vi "Color Sensor V3 Get CIE Yxy.vi"(8 "error in (no error)":errorcluster, 11 "ColorSensorDevRef":T1={"I2CDevRef"={"DevStatus"={"status"=FALSE, "code"=0, "source"=""}, "Device Address"=0, "Handle"=0, "I2C Bus"=enum."Invalid"}} {"I2CDevRef"."Device Address" format="%.0x"}) -> (0 "error out":errorcluster, 2 "CIE Yxy":cluster{"Yx":dbl, "Yy":dbl}, 3 "ColorSensorDevRef out":T1={"I2CDevRef"={"DevStatus"={"status"=FALSE, "code"=0, "source"=""}, "Device Address"=0, "Handle"=0, "I2C Bus"=enum."Invalid"}} {"I2CDevRef"."Device Address" format="%.0x"})   [LabVIEW 2023]
uses:
  Typedef/Color Sensor V3 DevRef.ctl
  <vilib>/Rock Robotics/WPI/I2C/WPI_I2CDevRef.ctl
  <vilib>/Rock Robotics/SystemInterfaces/i2clib/i2c_bus.ctl
  <vilib>/Analysis/Matrix/Datatypes/RealMatrix.ctl
  <vilib>/Analysis/baseanly.llb/Real A x B.vi
  <vilib>/Analysis/Matrix/NI_Matrix.lvlib
  <vilib>/Analysis/NI_AALBase.lvlib
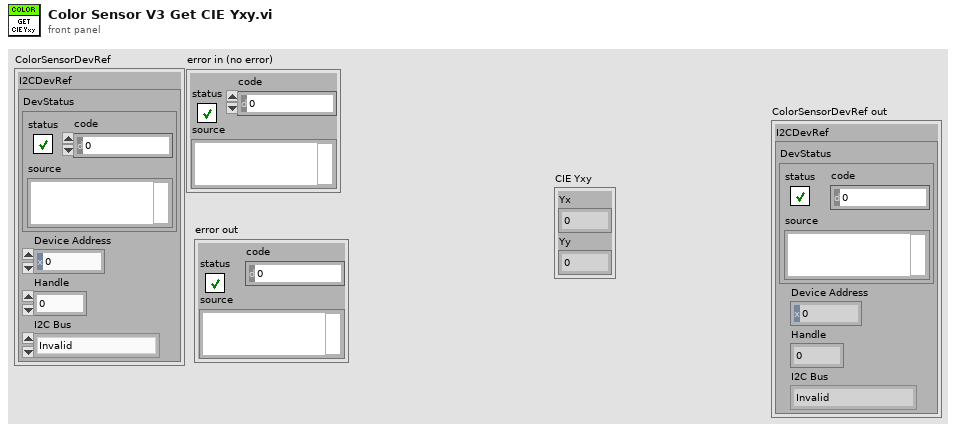
[diagram p1: front panel]
types:
  T1 = typedef "Color Sensor V3 DevRef.ctl" = cluster{"I2CDevRef":T2}
  T2 = typedef "WPI_I2CDevRef.ctl" = cluster{"DevStatus":errorcluster, "Device Address":u8, "Handle":i32, "I2C Bus":T3}
  T3 = typedef "i2c_bus.ctl" = enum16{"I2C On-Board", "I2C MXP", "Invalid"}
  T4 = typedef "NI_Matrix.lvlib/RealMatrix.ctl" = dbl[][]
  T5 = cluster{"Red":u32, "Green":u32, "Blue":u32, "IR":u32}
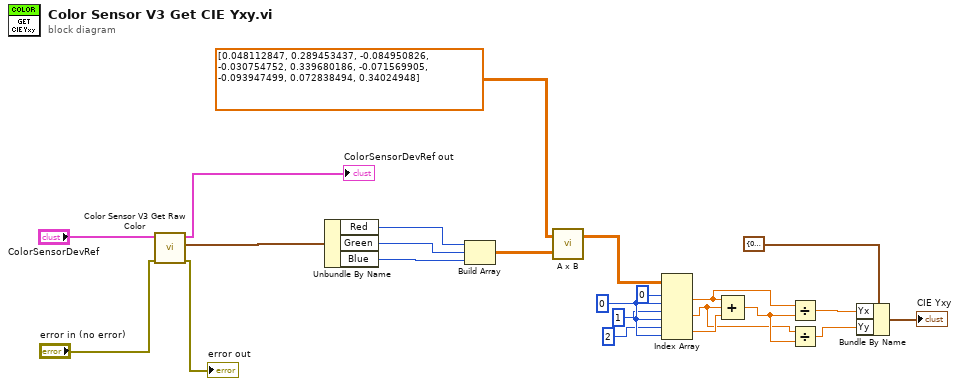
[diagram p0: block diagram]
diagram:
  w12 = 0 ("disabled index (col)")
  n1 = call "Color Sensor V3 Get Raw Color.vi"("error in (no error)"="error in (no error)", "ColorSensorDevRef"="ColorSensorDevRef") -> ("error out"=→"error out":errorcluster, "Raw Color"=w19:T5, "ColorSensorDevRef out"=→"ColorSensorDevRef out":T1)  [unwired: 7 in]
  n2 = Unbundle By Name(w19) -> ("Red"=w18:u32, "Green"=w17:u32, "Blue"=w16:u32)
  n3 = Build Array(w18, w17, w16) -> (w15:T4)
  n4 = call-poly <vilib>:"A x B.vi"("B"=w15, "A"=T4 [[0.048112847, 0.289453437, -0.084950826], [-0.030754752, 0.339680186, -0.071569905], [-0.093947499, 0.072838494, 0.34024948]] ("appended array")) -> ("A x B"=w13:T4)  [unwired: 1 out]
  n5 = Index Array(array=w13, index (row) #1=0 ("disabled index (col)"), index (col) #1=w12, index (row) #2=1 ("disabled index (col)"), index (col) #2=w12, index (row) #3=2 ("disabled index (col)"), index (col) #3=w12) -> (element #1=w3:dbl, element #2=w1:dbl, element #3=w8:dbl)
  n6 = Compound Arithmetic op=ADD(w3, w1, w8) -> (w2:dbl)
  n7 = Divide(x=w3, y=w2) -> (x/y=w5:dbl)
  n8 = Divide(x=w1, y=w2) -> (x/y=w4:dbl)
  n9 = Bundle By Name(cluster=cluster{"Yx":dbl, "Yy":dbl} {"Yx"=0.0, "Yy"=0.0} ("CIE Yxy"), "Yx"=w5, "Yy"=w4) -> (→"CIE Yxy":cluster{"Yx":dbl, "Yy":dbl})
